vi "MH_SetMarkerEdges.vi"(4 "me4":i32, 6 "me3":i32, 8 "error in (no error)":errorcluster, 9 "me2":i32, 10 "me1":i32, 11 "devidx":i32) -> (0 "error out":errorcluster, 3 "return type":i32)   [LabVIEW 2019]
uses:
  MH_DllPath_global.vi
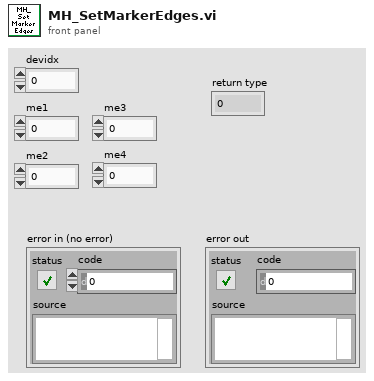
[diagram p1: front panel]
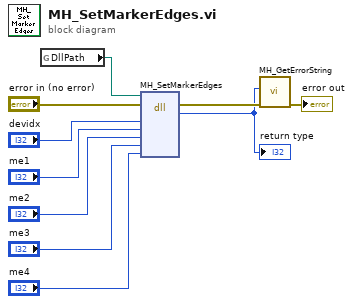
[diagram p0: block diagram]
diagram:
  n1 = global read "MH_DllPath_global.vi" "DllPath"() -> (w9:path)
  n2 = dll-call lib="MHLib64.dll" fn="MH_SetMarkerEdges"(path in=w9, error in="error in (no error)", "devidx"="devidx", "me1"="me1", "me2"="me2", "me3"="me3", "me4"="me4") -> (error out=w7:errorcluster, "return type"=w6:i32)  [unwired: 6 in, 1 out]
  "return type" <- w6
  n3 = call "MH_GetErrorString.vi"("error in (no error)"=w7, "code"=w6) -> ("error out"=→"error out":errorcluster)  [unwired: 7 in, 2 out]
